vi "Read Pressure Servo Settings.vi"(11 "PressureServoActuatorClosed in":refnum<class "PressureServoActuatorClosed.lvclass">) -> (2 "Pressure Servo Settings":T1={"Center Point"=413685.4733709468, "Area"=0.004536, "PA to PSI"=0.000145038, "Servo 1 DAC Channel"=1, "Servo 2 DAC Channel"=2, "Closed Loop Settings"={"P"=1.0, "I"=0.1, "D"=0.0, "Minimum"=0.0, "Maximum"=10.0}} {"Closed Loop Settings"."Maximum" format="%.4f"; "Closed Loop Settings"."Minimum" format="%.4f"; "Closed Loop Settings"."D" format="%.4f"; "Closed Loop Settings"."I" format="%.4f"; "Closed Loop Settings"."P" format="%.4f"; "Servo 2 DAC Channel" min=1 max=4 step=1; "Servo 1 DAC Channel" min=1 max=4 step=1; "PA to PSI" format="%.9f"; "Area" format="%.9f"; "Center Point" format="%.3f"}, 3 "PressureServoActuatorClosed out":refnum<class "PressureServoActuatorClosed.lvclass">)   [LabVIEW 2015, in "PressureServoActuatorClosed.lvclass"]
uses:
  PressureServoActuatorClosed.lvclass
  Typedefs/Pressure Servo Settings.ctl
  Typedefs/ClosedLoopSettings.ctl
  PressureServoActuatorClosed.lvclass/PressureServoActuatorClosed.ctl
  Typedefs/FAMTTypedefs.lvlib
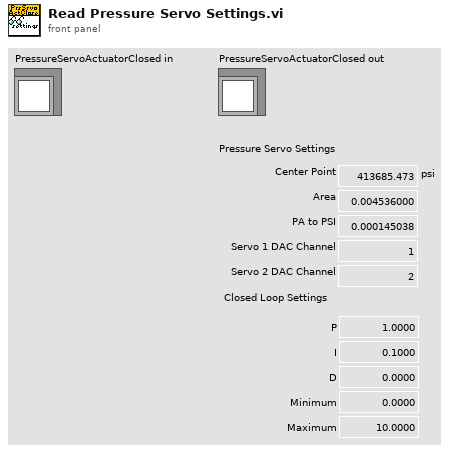
[diagram p1: front panel]
types:
  T1 = typedef "FAMTTypedefs.lvlib/Pressure Servo Settings.ctl" = cluster{"Center Point":dbl[unit], "Area":dbl, "PA to PSI":dbl, "Servo 1 DAC Channel":u8, "Servo 2 DAC Channel":u8, "Closed Loop Settings":T2}
  T2 = typedef "FAMTTypedefs.lvlib/ClosedLoopSettings.ctl" = cluster{"P":dbl, "I":dbl, "D":dbl, "Minimum":dbl, "Maximum":dbl}
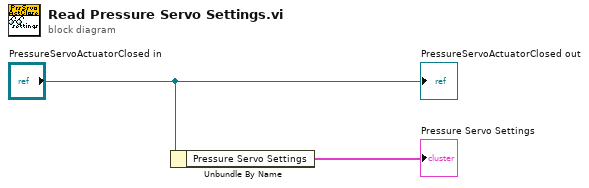
[diagram p0: block diagram]
diagram:
  n1 = Unbundle By Name("PressureServoActuatorClosed in") -> ("Pressure Servo Settings"=→"Pressure Servo Settings":T1)
  "PressureServoActuatorClosed out" <- "PressureServoActuatorClosed in"
